vi "DataBuffer2(SubVI).vi"(1 "Position":dbl[](array[numeric]), 2 "Bits":dbl[](array[numeric]), 3 "Buffer":dbl[][](array[numeric])) -> (0 "Data":dbl[][](array[numeric]))   [LabVIEW 2017]
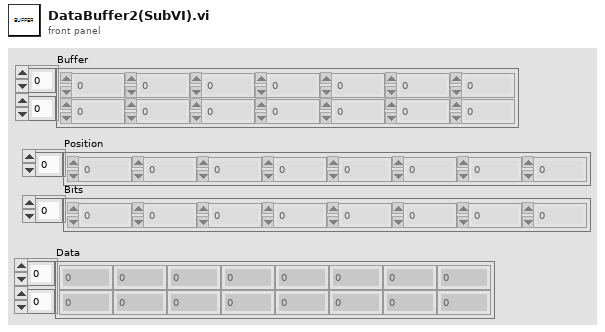
[diagram p1: front panel]
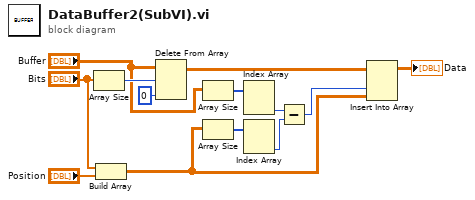
[diagram p0: block diagram]
diagram:
  n1 = Array Size(array="Bits") -> (size(s)=w13:i32)
  n2 = Build Array("Bits", "Position") -> (w5:dbl[][])
  n3 = Delete From Array(array="Buffer", length=w13, index (col)=0 ("비활성화된 인덱스 (열)")) -> (array with subset deleted=w8:dbl[][])  [unwired: 1 in, 1 out]
  n4 = Array Size(array="Buffer") -> (size(s)=w7:i32[])
  n5 = Array Size(array=w5) -> (size(s)=w6:i32[])
  n6 = Index Array(array=w7) -> (element #2=w4:i32)  [unwired: 2 in, 1 out]
  n7 = Index Array(array=w6) -> (element #2=w3:i32)  [unwired: 2 in, 1 out]
  n8 = Subtract(x=w4, y=w3) -> (x-y=w1:i32)
  n9 = Insert Into Array(array=w8, index (col)=w1, new element=w5) -> (→"Data":dbl[][])  [unwired: 1 in]
